vi "Runtime Test.vi"() -> ()   [LabVIEW 2015, in "PID Module tests.lvlib"]
doc: "This VI shows an example for how to test the Runtime functionality of the module. This will need to be modified according to module functionality."
uses:
  PID Module tests.lvlib
  module/execution/PID Module runtime.lvclass
  <vilib>/NI/Tag Bus/dictionary/data dictionary.lvclass/data dictionary.ctl
  <vilib>/NI/Tag Bus/dictionary/lookup polymorphs/locate double.vi
  <vilib>/NI/Tag Bus/table/data polymorphs/write one/write Double.vi
  <vilib>/NI/Tag Bus/table/data polymorphs/read one/read Double.vi
  <vilib>/NI/Tag Bus/dictionary/search/find data index.vi
  <vilib>/NI/Tag Bus/dictionary/search/search string list.vi
  <vilib>/NI/Tag Bus/dictionary/tag not found.vi
  module/configuration/PID Module configuration.lvclass
  <vilib>/NI/Tag Bus/dictionary/data dictionary.lvclass
  <vilib>/NI/Tag Bus/table/data table.lvlib
panel:
  in  "stop":bool
  in  "Variable":dbl
  out "Ouput":dbl
  in  "Setpoint":dbl
  out "error":errorcluster
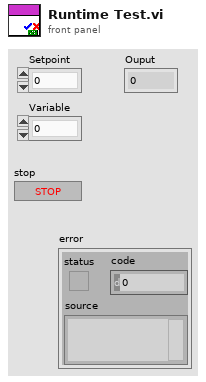
[diagram p1: front panel]
types:
  T1 = typedef "TBM channel.lvclass/data tables.ctl" = cluster{"input data":T2, "processing parameter":T2, "processing result":T2, "output data":T2}
  T2 = typedef "tag bus.lvlib/dictionary table pair.ctl" = cluster{"data dictionary":refnum<class "data dictionary.lvclass">, "data table":T3}
  T3 = typedef "tag bus.lvlib/data table.lvlib/data table.ctl" = cluster{"Double":dbl[], "Single":sgl[], "I64":i64[], "I32":i32[], "I16":i16[], "I8":i8[], "U64":u64[], "U32":u32[], "U16":u16[], "U8":u8[], "Boolean":bool[], "String":string[], "Array of Double":cluster{"DBL Array":dbl[]}[], "Array of Single":cluster{"SGL Array":sgl[]}[], "Array of I64":cluster{"I64 Array":i64[]}[], "Array of I32":cluster{"I32 Array":i32[]}[], "Array of I16":cluster{"I16 Array":i16[]}[], "Array of I8":cluster{"I8 Array":i8[]}[], "Array of U64":cluster{"U64 Array":u64[]}[], "Array of U32":cluster{"U32 Array":u32[]}[], "Array of U16":cluster{"U16 Array":u16[]}[], "Array of U8":cluster{"U8 Array":u8[]}[], "Array of Boolean":cluster{"Boolean Array":bool[]}[], "Array of String":cluster{"String Array":string[]}[]}
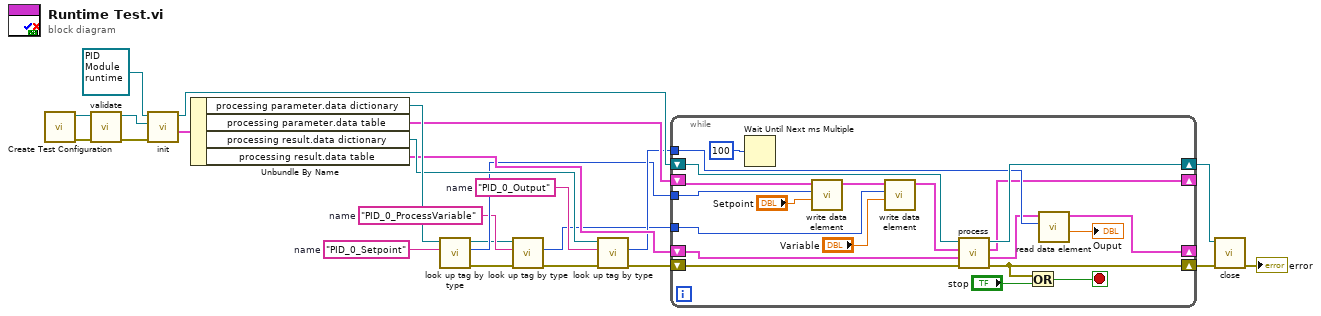
[diagram p0: block diagram]
diagram:
  w7 = "PID_0_Setpoint"  # name
  w6 = "PID_0_ProcessVariable"  # name
  w10 = "PID_0_Output"  # name
  n1 = call "Create Test Configuration.vi"() -> ("error out"=w20:errorcluster, "Module Configuration"=w21:refnum<class "PID Module configuration.lvclass">)  [unwired: 6 in, 4 out]
  n2 = call-dynamic "validate.vi"("error in"=w20, "PID Module 2 configuration in"=w21) -> ("error out"=w23:errorcluster, "PID Module 2 configuration out"=w22:refnum<class "PID Module configuration.lvclass">)  [unwired: 8 in]
  n3 = call-dynamic "init.vi"("error in"=w23, "TBM module configuration in"=w22, "PID Module 2 runtime in"=refnum<class "PID Module runtime.lvclass"> refnum ("tag bus configurable plugin module")) -> ("data allocations"=w13:T1, "PID Module 2 runtime out"=w14:refnum<class "PID Module runtime.lvclass">)  [unwired: 5 in, 2 out]
  n4 = Unbundle By Name(w13) -> ("processing parameter.data dictionary"=w19:refnum<class "data dictionary.lvclass">, "processing parameter.data table"=w18:T3, "processing result.data dictionary"=w16:refnum<class "data dictionary.lvclass">, "processing result.data table"=w15:T3)
  n5 = call-poly <vilib>:"look up tag by type.vi"("name"=w7, "data dictionary in"=w19) -> ("error out"=w3:errorcluster, "index"=w9:i32, "data dictionary out"=w4:refnum<class "data dictionary.lvclass">)  [unwired: 7 in]
  n6 = call-poly <vilib>:"look up tag by type.vi"("error in"=w3, "name"=w6, "data dictionary in"=w4) -> ("error out"=w2:errorcluster, "index"=w5:i32)  [unwired: 6 in, 1 out]
  n7 = call-poly <vilib>:"look up tag by type.vi"("error in"=w2, "name"=w10, "data dictionary in"=w16) -> ("error out"=w1:errorcluster, "index"=w11:i32)  [unwired: 6 in, 1 out]
  n8 = while {
    tunnel: w11 -> [w40]
    tunnel: w9 -> [w39]
    tunnel: w5 -> [w33]
    shift-right: [w41] -> w12
    shift-left: w14 -> [w42]
    shift-right: [w27] -> w8
    shift-left: w1 -> [w31]
    shift-right: [w26] -> _
    shift-left: w18 -> [w44]
    shift-right: [w25] -> _
    shift-left: w15 -> [w43]
    stop <- w28 stop-if-true
    n9 = Wait Until Next ms Multiple(millisecond multiple=u32 100) -> ()  [unwired: 1 out]
    n10 = call-poly <vilib>:"write data element.vi"("value"="Setpoint", "index"=w39, "data table in"=w44) -> ("data table out"=w34:T3)  [unwired: 8 in]
    n11 = call-poly <vilib>:"write data element.vi"("value"="Variable", "index"=w33, "data table in"=w34) -> ("data table out"=w32:T3)  [unwired: 8 in]
    n12 = call-dynamic "process.vi"("error in"=w31, "result allocation"=w43, "parameters"=w32, "module in"=w42) -> ("error out"=w27:errorcluster, "results"=w38:T3, "parameter allocation"=w26:T3, "module out"=w41:refnum<class "PID Module runtime.lvclass">)  [unwired: 4 in]
    n13 = Or(x=w27, y="stop") -> (x .or. y?=w28:bool)
    n14 = call-poly <vilib>:"read data element.vi"("index"=w40, "data table in"=w38) -> ("value"=→"Ouput":dbl, "data table out"=w25:T3)  [unwired: 8 in]
  }
  n15 = call-dynamic "close.vi"("error in"=w8, "PID Module 2 runtime in"=w12) -> ("error out"=→"error":errorcluster)  [unwired: 9 in]
